vi "PCS Correlation.vi"() -> ()   [LabVIEW 2022 SP3]
uses:
  <vilib>/Analysis/baseanly.llb/Mean (DBL).vi
  <vilib>/Utility/file.llb/Read From Spreadsheet File (DBL).vi
  <vilib>/Analysis/NI_AALBase.lvlib
panel:
  out "Cumulant ln fit":cluster{"Time":dbl[], "ln(x)":dbl[]}[](graph)
  out "aurocorrelation":T1(graph)
  out "Cumulant Fit":T2
  out "Fit":T3
  out "SVM Gaps":cluster{i32, "x":i32, dbl[][]}(graph)
  out "SVM Size (um)":cluster{i32, "x":i32, dbl[][]}(graph)
  out "SVM Fit to column data":T3
  in  "New File":bool
  out "File Path":path
  in  "Save Bin Data":bool
  in  "Data Source":enum16{"Thor File", "NI Card Grab", "NI File"}(ring)=enum."NI Card Grab"
  in  "AC length":i32=500
  in  "Capture Bins":i32=2097153
  out "Time step (ms)":dbl
  in  "zero lag +":i32=1
  in  "Sample Rate (Hz)":dbl=100000.0
  in  "counts per bin":dbl[](graph)
  out "mean":dbl format="%0.2f"
  out "Theory":T4
  in  "Diameter (um)":dbl=0.04
  # "Expected decay"
  # "`"
  # "Raw G2 Fit"
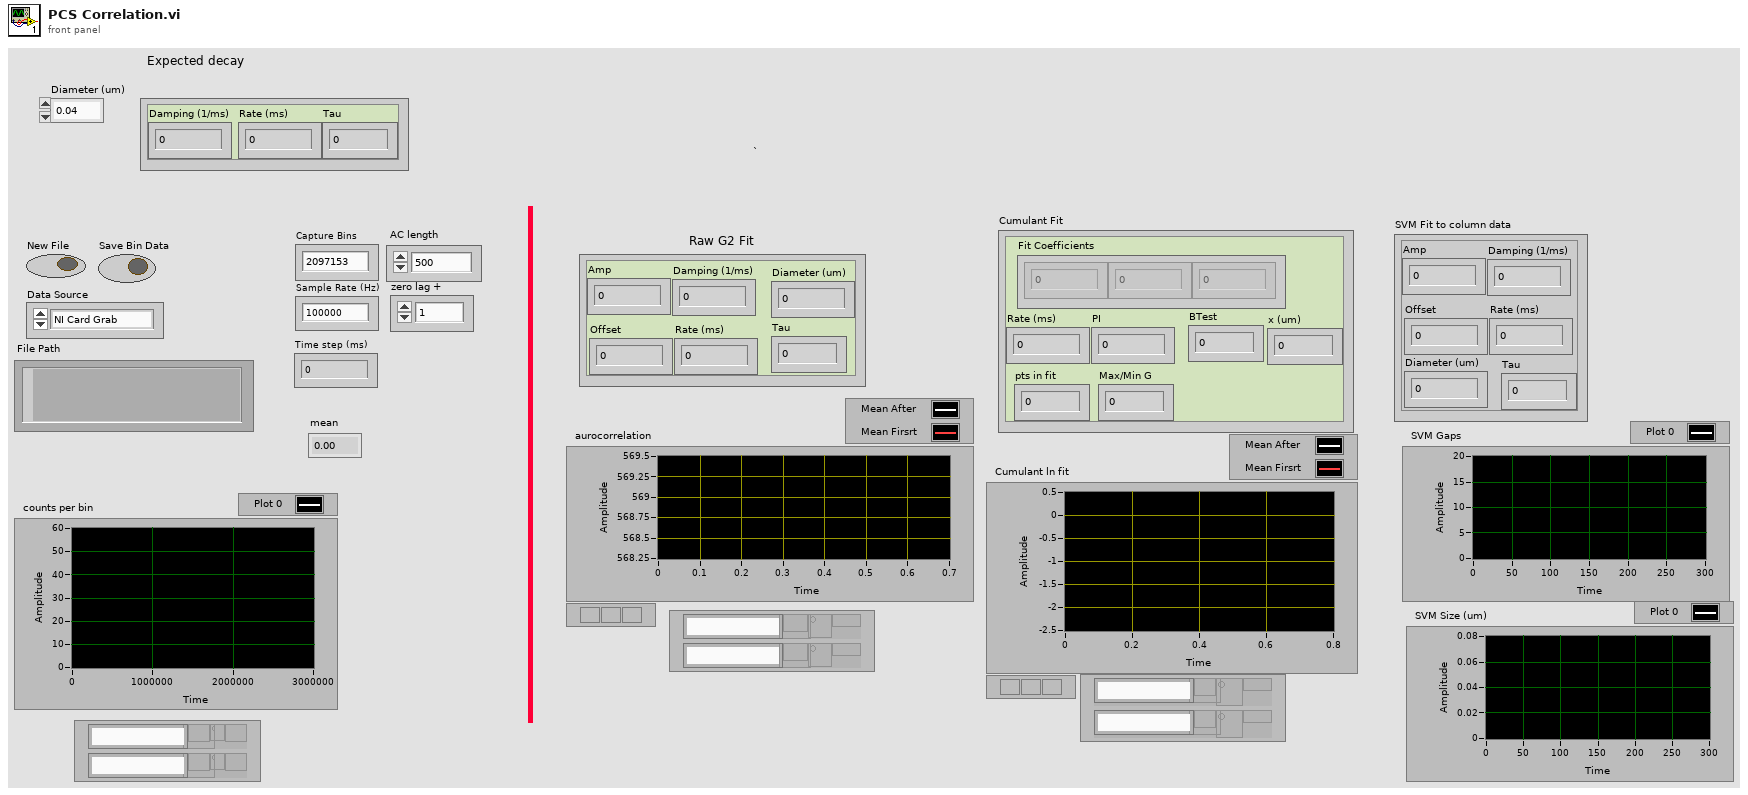
[diagram p1: front panel]
types:
  T1 = cluster{"Time":dbl[], "Best Exponential Fit":dbl[]}[]
  T2 = cluster{"Fit Coefficients":dbl[], "Rate (ms)":dbl, "PI":dbl, "BTest":dbl, "x (um)":dbl, "pts in fit":dbl, "Max/Min G":dbl}
  T3 = cluster{"Amp":dbl, "Offset":dbl, "Damping (1/ms)":dbl, "Rate (ms)":dbl, "Diameter (um)":dbl, "Tau":dbl}
  T4 = cluster{"Damping (1/ms)":dbl, "Rate (ms)":dbl, "Tau":dbl}
  T5 = enum16{"open", "replace", "create", "open or create", "replace or create", "replace or create with confirmation"}
  T6 = enum16{"big-endian, network order", "native, host order", "little-endian"}
  T7 = cluster{"Amp":dbl, "Offset":dbl, "Damping (1/ms)":dbl, "Rate (ms)":dbl, "Diameter (um)":dbl, "Tau":dbl}[][]
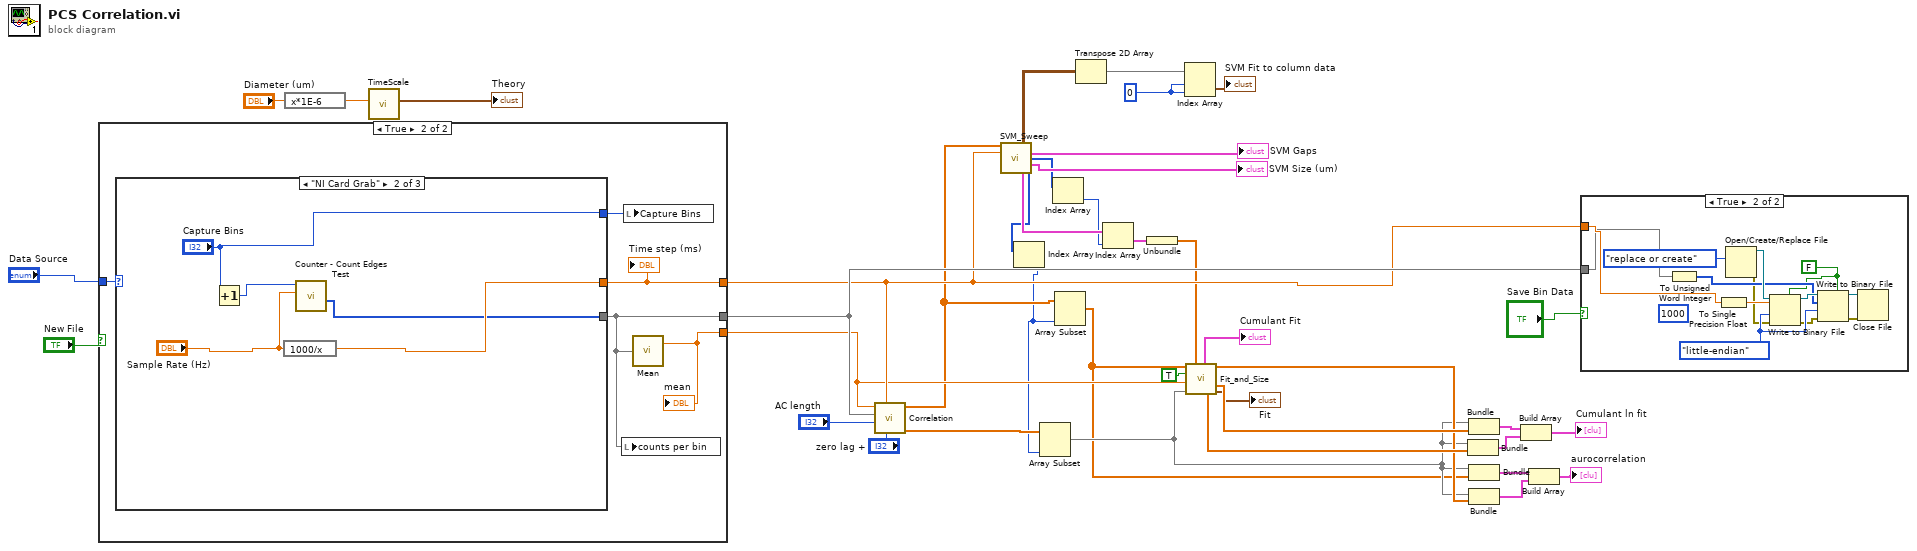
[diagram p0: block diagram]
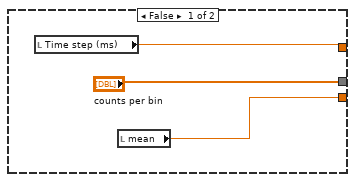
[diagram p2: hidden frame]
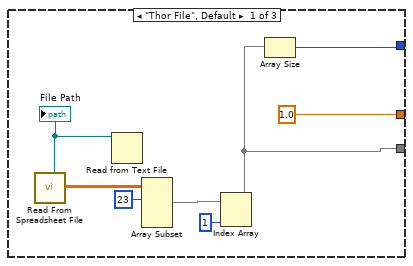
[diagram p3: hidden frame]
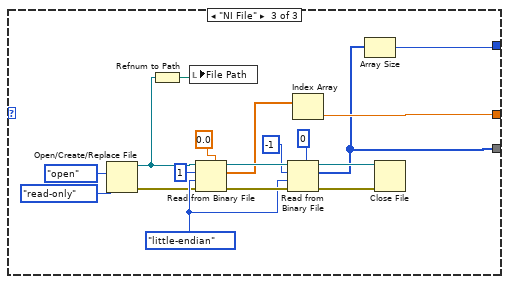
[diagram p4: hidden frame]
diagram:
  w4 = 0 ("disabled index (col)")
  n1 = case shown="True" "New File" {
    tunnel: ["counts per bin" w44] -> w35
    tunnel: [w43 w47] -> w21
    tunnel: "Data Source" -> [_ w48]
    tunnel: [w41 w45] -> w20
    frame False {
      n2 = local read "Time step (ms)"() -> (w43:dbl)
      n3 = local read "mean"() -> (w41:dbl)
    }
    frame True {
      n4 = case shown="\"NI Card Grab\"" w48 {
        tunnel: [w49 w57 w62] -> w44
        tunnel: [1.0 ("Time step (ms)") w60 w69] -> w47
        tunnel: [w50 "Capture Bins" w66] -> w46
        frame "Thor File", Default {
          n5 = call-poly <vilib>:"Read From Spreadsheet File.vi"() -> ("all rows"=w54:dbl[][], "new file path (Not A Path if cancelled)"=w53:path)  [unwired: 7 in, 3 out]
          "File Path" <- w53
          n6 = Read from Text File(file (use dialog)=w53) -> ()  [unwired: 3 in, 4 out]
          n7 = Array Subset(array=w54, index (row)=23 ("index")) -> (w51:dbl[][])  [unwired: 3 in]
          n8 = Index Array(array=w51, index (col)=1 ("disabled index (col)")) -> (element=w49:dbl[])  [unwired: 1 in]
          n9 = Array Size(array=w49) -> (size(s)=w50:i32)
        }
        frame "NI Card Grab" {
          n10 = Increment(x="Capture Bins") -> (x+1=w59:i32)
          n11 = expression code="1000/x"("Sample Rate (Hz)") -> (w60:dbl)
          n12 = call "Counter - Count Edges Test.vi"("Sample Rate"="Sample Rate (Hz)", "Samples per Loop"=w59) -> ("counts/bin"=w57:u32[])  [unwired: 8 in, 1 out]
        }
        frame "NI File" {
          w76 = T6."little-endian" ("byte order (0:big-endian, network order)")
          n13 = Open/Create/Replace File(operation (0:open)=T5."open", access (0:read/write)=enum16{"read/write", "read-only", "write-only"}."read-only") -> (refnum out=w65:refnum<file>, error out=w73:errorcluster)  [unwired: 4 in, 1 out]
          n14 = Refnum to Path(1:w65) -> (0:w64:path)
          n15 = local write "File Path"(w64) -> ()
          n16 = Read from Binary File(5:sgl 0.0, 8:w73, 9:w76, 10:1 ("count (1)"), 11:w65) -> (0:w77:errorcluster, 2:w68:sgl[], 3:w78:refnum<file>)  [unwired: 1 in, 1 out]
          n17 = Read from Binary File(5:u16 0, 8:w77, 9:w76, 10:-1 ("count (1)"), 11:w78) -> (0:w63:errorcluster, 2:w62:u16[], 3:w72:refnum<file>)  [unwired: 1 in, 1 out]
          n18 = Index Array(array=w68) -> (element=w69:sgl)  [unwired: 1 in]
          n19 = Array Size(array=w62) -> (size(s)=w66:i32)
          n20 = Close File(refnum=w72, error in=w63) -> ()  [unwired: 2 out]
        }
      }
      "Time step (ms)" <- w47
      n21 = local write "counts per bin"(w44) -> ()
      n22 = local write "Capture Bins"(w46) -> ()
      n23 = call-poly <vilib>:"Mean.vi"("X"=w44) -> ("mean"=w45:dbl)  [unwired: 1 out]
      "mean" <- w45
    }
  }
  n24 = expression code="x*1E-6"("Diameter (um)") -> (w39:dbl)
  n25 = call "TimeScale.vi"("Diameter (m)"=w39) -> ("Theory"=→"Theory":T4)  [unwired: 10 in]
  n26 = call "Correlation.vi"("zero lag +"="zero lag +", "Time step (ms)"=w21, "AC final pts"="AC length", "counts/bin"=w35, "mean"=w20) -> ("Time"=w12:dbl[], "Data out"=w14:dbl[])  [unwired: 5 in]
  n27 = call "SVM_Sweep.vi"("Data IN"=w14, "time step"=w21) -> ("SVM Out Stack"=w18:T7, "SV Gaps"=→"SVM Gaps":cluster{i32, "x":i32, dbl[][]}, "Max Index"=w3:i32[], "SVM Size (um)"=→"SVM Size (um)":cluster{i32, "x":i32, dbl[][]}, "Array"=w15:cluster{"A tau":dbl[]}[], "Best Size"=w8:i32[])  [unwired: 6 in, 2 out]
  n28 = Index Array(array=w8) -> (element=w7:i32)  [unwired: 1 in]
  n29 = Array Subset(array=w12, length=w7) -> (w11:dbl[])  [unwired: 1 in]
  n30 = Index Array(array=w3) -> (element=w1:i32)  [unwired: 1 in]
  n31 = Array Subset(array=w14, length=w7) -> (w10:dbl[])  [unwired: 1 in]
  n32 = Transpose 2D Array(2D array=w18) -> (transposed array=w2:T7)
  n33 = Index Array(array=w15, index=w1) -> (element=w16:cluster{"A tau":dbl[]})
  n34 = Unbundle(w16) -> ("A tau"=w13:dbl[])
  n35 = Index Array(array=w2, index (row)=w4, index (col)=w4) -> (element=→"SVM Fit to column data":T3)
  n36 = call "Fit_and_Size.vi"("G2"=w10, "A tau"=w13, "A(tau)"=TRUE, "bin mean"=w20, "Time"=w11) -> ("Cumulant Fit"=→"Cumulant Fit":T2, "Best Exponential Fit"=w27:dbl[], "Best Polynomial Fit"=w32:dbl[], "ln(x)/2"=w31:dbl[], "Fit"=→"Fit":T3)  [unwired: 5 in, 1 out]
  n37 = Bundle(w11, "ln(x)/2"=w31) -> (w29:cluster{dbl[], "ln(x)/2":dbl[]})  [unwired: 1 in]
  n38 = Bundle(w11, "Best Polynomial Fit"=w32) -> (w30:cluster{dbl[], "Best Polynomial Fit":dbl[]})  [unwired: 1 in]
  n39 = Bundle(w11, w10) -> (w25:cluster{dbl[], dbl[]})  [unwired: 1 in]
  n40 = Bundle(w11, "Best Exponential Fit"=w27) -> (w26:cluster{dbl[], "Best Exponential Fit":dbl[]})  [unwired: 1 in]
  n41 = Build Array(w30, w29) -> (→"Cumulant ln fit":cluster{dbl[], "ln(x)/2":dbl[]}[])
  n42 = Build Array(w25, w26) -> (→"aurocorrelation":cluster{dbl[], "Best Exponential Fit":dbl[]}[])
  n43 = case shown="True" "Save Bin Data" {
    tunnel: w35 -> [_ w88]
    tunnel: w21 -> [_ w92]
    frame False {
    }
    frame True {
      w84 = FALSE ("prepend array or string size? (T)")
      w86 = T6."little-endian" ("byte order (0:big-endian, network order)")
      (unwired) 1000
      n44 = To Unsigned Word Integer(number=w88) -> (unsigned 16bit integer=w87:u16[])
      n45 = To Single Precision Float(number=w92) -> (single precision float=w91:sgl)
      n46 = Open/Create/Replace File(operation (0:open)=T5."replace or create") -> (refnum out=w90:refnum<file>, error out=w80:errorcluster)  [unwired: 5 in, 1 out]
      n47 = Write to Binary File(file (use dialog)=w90, data=w91, error in=w80, 5:w84, 9:w86) -> (refnum out=w89:refnum<file>, error out=w85:errorcluster)  [unwired: 1 in, 1 out]
      n48 = Write to Binary File(file (use dialog)=w89, data=w87, error in=w85, 5:w84, 9:w86) -> (refnum out=w82:refnum<file>, error out=w83:errorcluster)  [unwired: 1 in, 1 out]
      n49 = Close File(refnum=w82, error in=w83) -> ()  [unwired: 2 out]
    }
  }
